vi "sub_uniform_filter.vi"(8 "Uniform window":i32=3, 11 "Input 1D array":dbl[](array[numeric])) -> (3 "filtered 1D array":dbl[](array[numeric]))   [LabVIEW 2020]
uses:
  <vilib>/imath/engines/lvmath2/RunTimeEngine/Managers/WorkSpace/UID Generator.vi
  <vilib>/imath/engines/lvmath2/RunTimeEngine/BuiltInFunctions/ones/NIMS_V=ones(I32,I32).vi
  <vilib>/imathl/engines/lvmath/Functions/Error Handling/Create Error.vi
  <vilib>/imath/engines/lvmath2/RunTimeEngine/BuiltInFunctions/filter/NIMS_filter(GV,GV,GV,GV,Str).vi
  <instcachedir>/0/NIMS_filter(GV,GV,GV,GV,Str)_4B685211BB584ED18C643EEF72E0E7AA.lvgen/NIMS_filter(GV,GV,GV,GV,Str)_4B685211BB584ED18C643EEF72E0E7AA_000.vi
  <vilib>/imath/engines/lvmath2/RunTimeEngine/RunTimeType/NIMS_RunTimeType_From StrictType (excl LVString).vi
  <instcachedir>/0/NIMS_RunTimeType_From StrictType (excl LVString)_867E31CEF7BF4ABF8B0CFC3D01EB2647.lvgen/NIMS_RunTimeType_From StrictType (excl LVString)_867E31CEF7BF4ABF8B0CFC3D01EB2647_000.vi
  <vilib>/imath/engines/lvmath2/RunTimeEngine/LocalVariableDefStatement/MC_LocalVariableDefStatement_Display.vi
  <vilib>/imath/engines/lvmath2/RunTimeEngine/Managers/SymbolTable/Clear UID.vi
  <vilib>/imath/engines/lvmath2/RunTimeEngine/NodeEndStatement/NIMS_NodeEndStatement_Output.vi
  <instcachedir>/0/NIMS_NodeEndStatement_Output_53EC0D466D134D7ABD903AC30B43404B.lvgen/NIMS_NodeEndStatement_Output_53EC0D466D134D7ABD903AC30B43404B_005.vi
  <vilib>/imath/engines/lvmath2/RunTimeEngine/ErrorHandling/NIMS_Finalize Error.vi
  <vilib>/imath/engines/lvmath2/RunTimeEngine/Managers/SymbolTable/NIMS_WorkSpace.lvlib
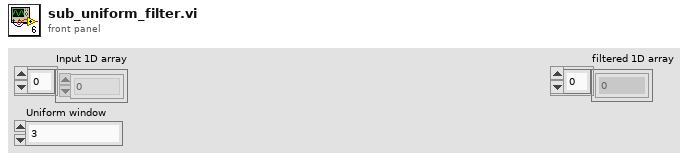
[diagram p1: front panel]
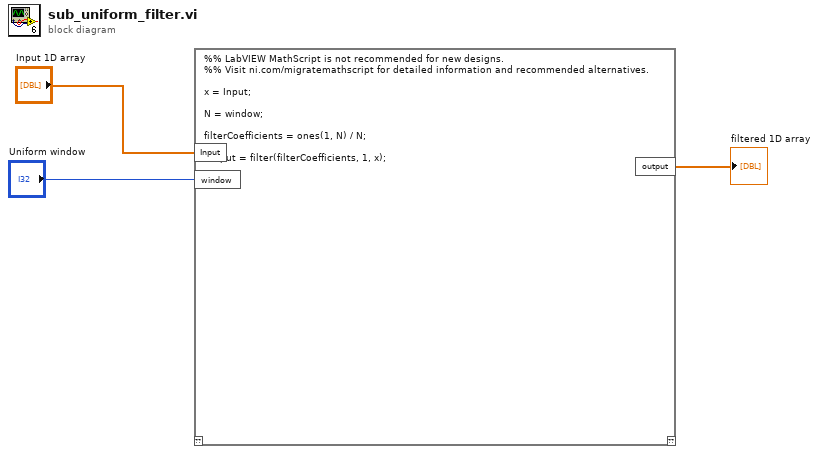
[diagram p0: block diagram]
diagram:
  n1 = mathscript code="%% LabVIEW MathScript is not recommended for new designs.\n%% Visit ni.com/migratemathscript for detailed information and recommended alternatives.\n\nx = Input;\n\nN = window;\n\nfilterCoefficients = ones(1, N) / N;\n\noutput = filter(filterCoefficients, 1, x);\n\noutput"("Input"="Input 1D array", "window"="Uniform window") -> ("output"=→"filtered 1D array":dbl[])  [unwired: 1 in, 1 out]
